vi "Write Armed Response Synchronizer.vi"(8 "error in (no error)":errorcluster, 10 "Response Synchronizer.lvclass":refnum<class "Response Synchronizer.lvclass">, 11 "Pulse Controller in":refnum<class "Pulse Controller.lvclass">) -> (0 "error out":errorcluster, 3 "Pulse Controller out":refnum<class "Pulse Controller.lvclass">)   [LabVIEW 2021, in "Pulse Controller.lvclass"]
uses:
  Pulse Controller.lvclass
  Pulse Controller.lvclass/Pulse Controller.ctl
  NHMFL_Core/Libraries/Instruments/Results/Response Synchronizer/Response Synchronizer.lvclass
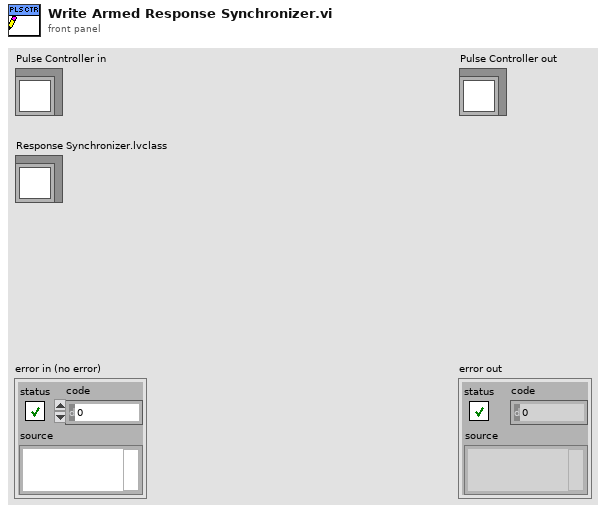
[diagram p1: front panel]
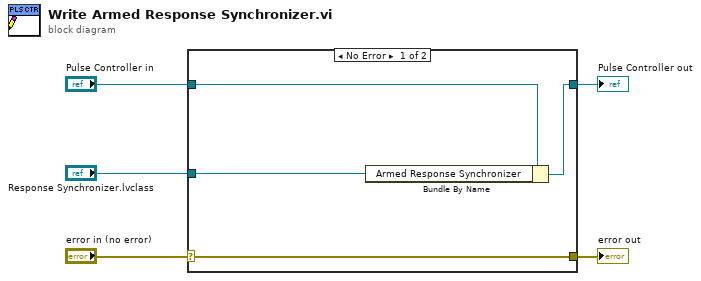
[diagram p0: block diagram]
diagram:
  n1 = case shown="No Error" "error in (no error)" {
    selector: "error in (no error)" -> [w9 w10]
    tunnel: [w9 w10] -> w4
    tunnel: [w7 w11] -> w2
    tunnel: "Pulse Controller in" -> [w8 w11]
    tunnel: "Response Synchronizer.lvclass" -> [w6 _]
    frame No Error {
      n2 = Bundle By Name(cluster=w8, "Armed Response Synchronizer"=w6) -> (w7:refnum<class "Pulse Controller.lvclass">)
    }
    frame Error {
    }
  }
  "error out" <- w4
  "Pulse Controller out" <- w2
